vi "Flow Velocity Calculator.vi"() -> ()   [LabVIEW 2024]
uses:
  <vilib>/numeric/Random Number (Range) DBL.vi
  <vilib>/Instr/_visa.llb/VISA Configure Serial Port (Instr).vi
panel:
  out "appended array":string[][](array[string])
  out "Density":dbl
  out "read buffer":string
  in  "stop":bool
  out "sqrt(x)":dbl
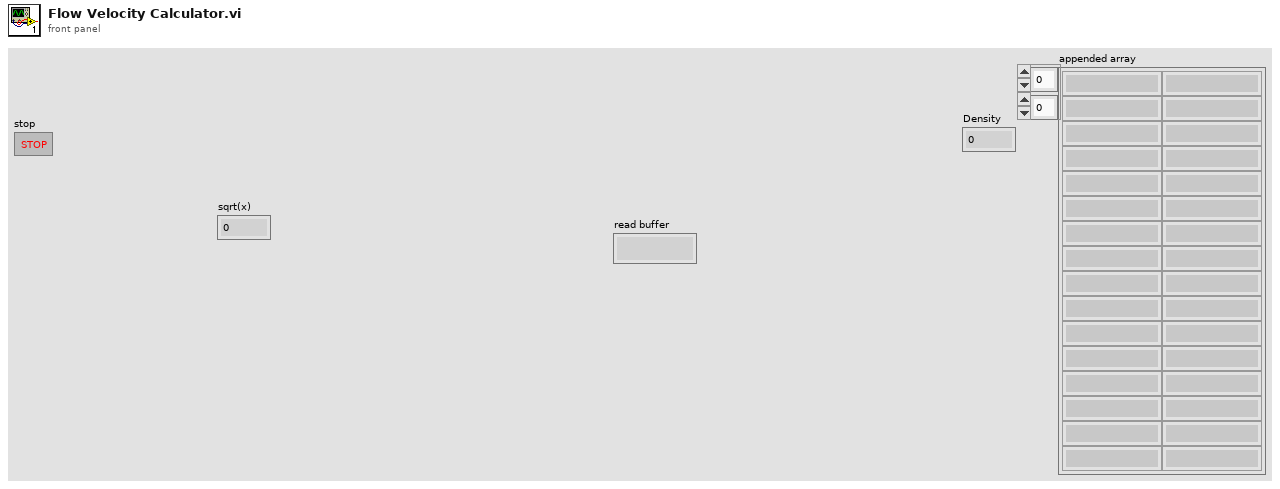
[diagram p1: front panel]
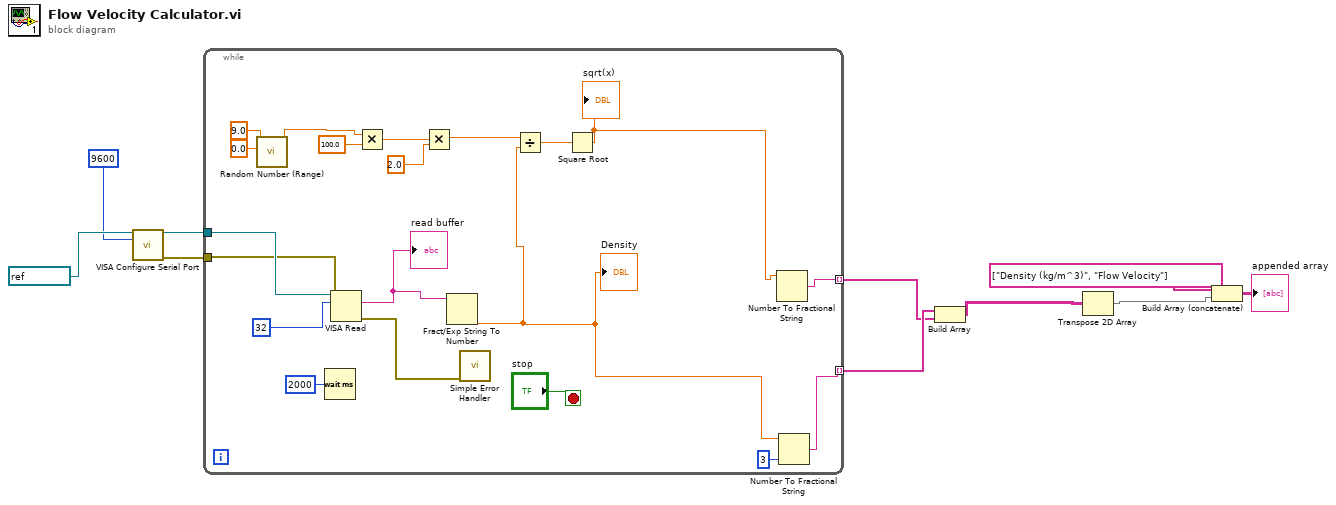
[diagram p0: block diagram]
diagram:
  n1 = call-poly "VISA Configure Serial Port"("VISA resource name"=refnum<visa-resource-name> "COM5", "baud rate (9600)"=u32 9600) -> ("VISA resource name out"=w8:refnum<visa-resource-name>, "error out"=w7:errorcluster)  [unwired: 12 in]
  n2 = while {
    tunnel: w8 -> [w30]
    tunnel: w7 -> [w29]
    tunnel: [w12] -> w5 mode=indexing
    tunnel: [w14] -> w6 mode=indexing
    stop <- "stop" stop-if-true
    n3 = call-poly <vilib>:"Random Number (Range).vi"("lower bound (0)"=0.0, "upper bound (100)"=9.0) -> ("number"=w21:dbl)  [unwired: 9 in]
    n4 = Wait (ms)(milliseconds to wait=u32 2000) -> ()  [unwired: 1 out]
    n5 = VISA Read(VISA resource name=w30, byte count=u32 32, error in (no error)=w29) -> (read buffer=w16:string, error out=w28:errorcluster)  [unwired: 2 out]
    "read buffer" <- w16
    n6 = Multiply(x=w21, y=100.0) -> (x*y=w22:dbl)
    n7 = Multiply(x=w22, y=2.0) -> (x*y=w24:dbl)
    n8 = Fract/Exp String To Number(string=w16) -> (number=w15:dbl)  [unwired: 3 in, 1 out]
    "Density" <- w15
    n9 = call <vilib>:"Simple Error Handler.vi"("error in (no error)"=w28) -> ()  [unwired: 4 in, 5 out]
    n10 = Divide(x=w24, y=w15) -> (x/y=w23:dbl)
    n11 = Square Root(x=w23) -> (sqrt(x)=w13:dbl)
    "sqrt(x)" <- w13
    n12 = Number To Fractional String(number=w13) -> (F-format string=w12:string)  [unwired: 3 in]
    n13 = Number To Fractional String(number=w15, precision (6)=i16 3) -> (F-format string=w14:string)  [unwired: 2 in]
  }
  n14 = Build Array(w6, w5) -> (w4:string[][])
  n15 = Transpose 2D Array(2D array=w4) -> (transposed array=w2:string[][])
  n16 = Build Array (concatenate)(string[] ["Density (kg/m^3)", "Flow Velocity"], w2) -> (→"appended array":string[][])
